vi "VCL_2_DSC_BATCH.vi"(8 "error in (no error)":errorcluster, 11 "path to logfile or directory":path) -> (0 "error out":errorcluster)   [LabVIEW 2016, in "VCL_2_DSC.lvclass"]
uses:
  VCL_2_DSC.lvclass
  typedefs/write-enum.ctl
  <vilib>/addons/WireFlow/_WF_ProgressBar.llb/ProgressBar_WireFlow.lvclass
panel:
  in  "Enum":T1
  in  "Process":bool
  in  "STOP":bool
  out "standard output":string
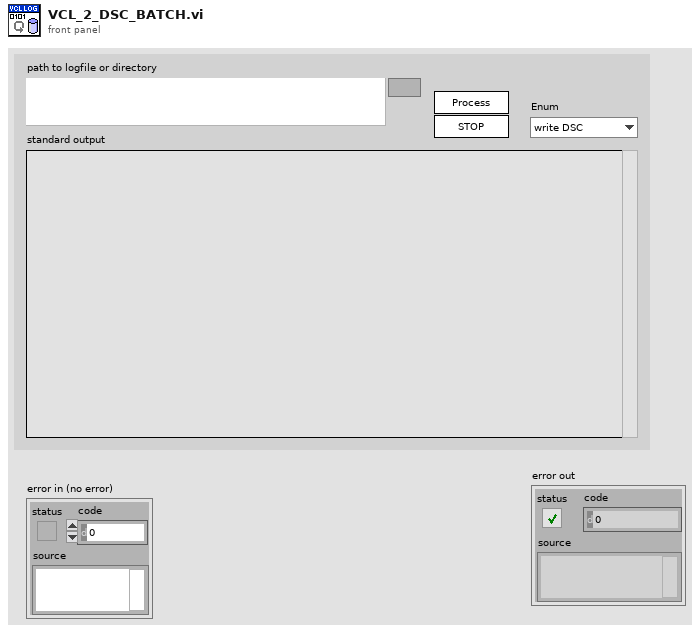
[diagram p1: front panel]
types:
  T1 = typedef "VCL_2_DSC.lvclass/write-enum.ctl" = enum16{"write DSC", "write TDMS", "no write"}
  T2 = enum32{"invalid app kind", "Development System", "Run Time System", "Student Edition", "Embedded LabVIEW", "Evaluation", "Custom"}
  T3 = enum32{"Invalid", "Standard", "Closed", "Hidden", "Minimized", "Maximized"}
  T4 = cluster{"Core":cluster{"Current VI Reference":refnum<vi>, "Close Panel on Exit?":bool}, "vcl paths":path[], "txt paths":path[], "WF-ProgressBar":refnum<class "ProgressBar_WireFlow.lvclass">}
  T5 = cluster{"Current VI Reference":refnum<vi>, "Close Panel on Exit?":bool}
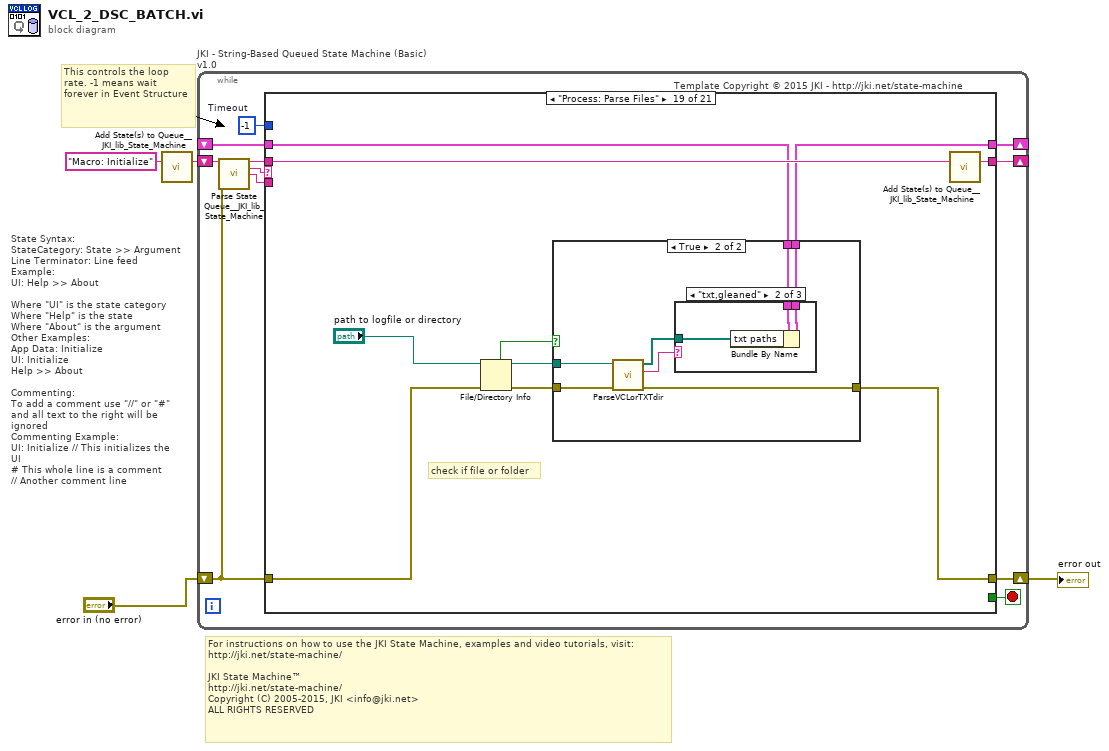
[diagram p0: block diagram]
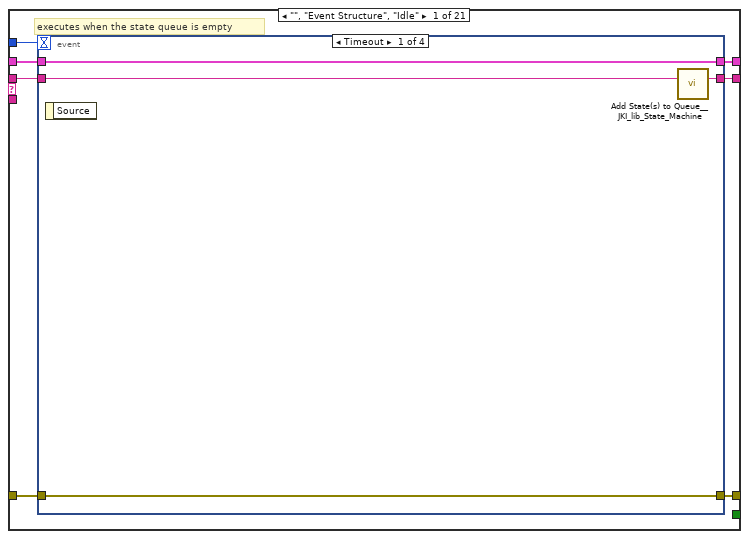
[diagram p2: hidden frame]
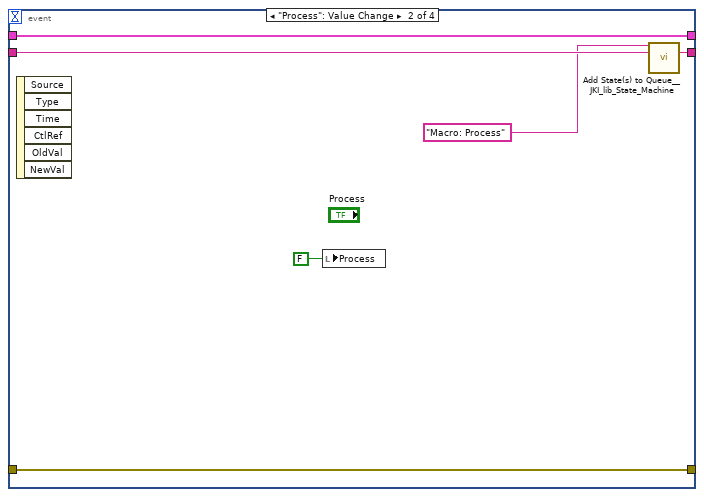
[diagram p3: hidden frame]
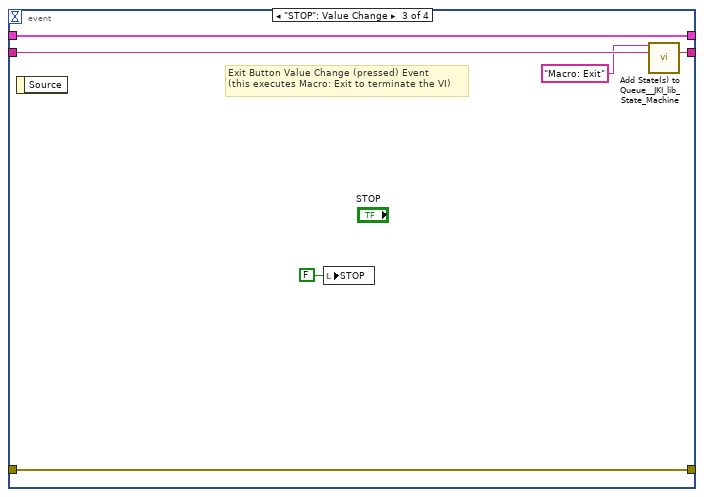
[diagram p4: hidden frame]
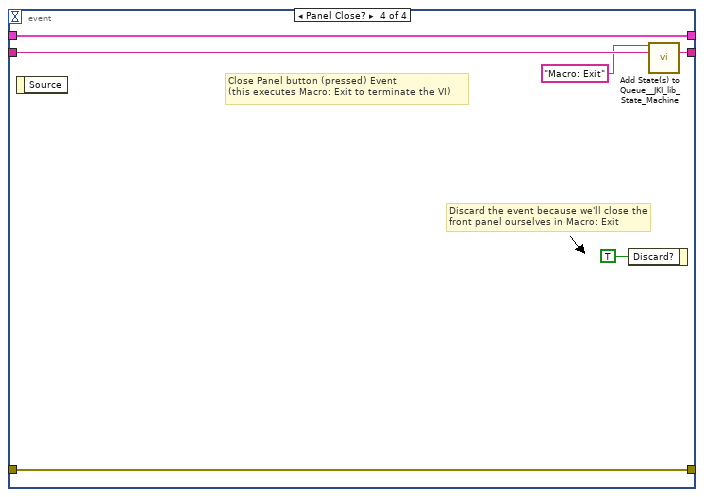
[diagram p5: hidden frame]
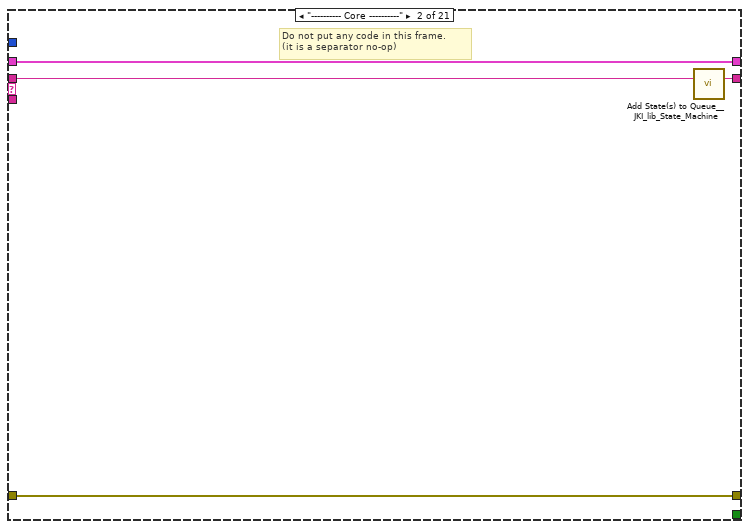
[diagram p6: hidden frame]
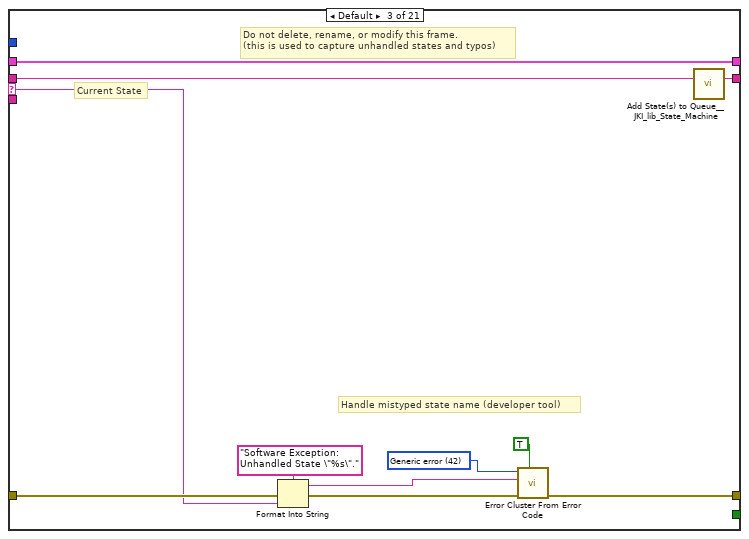
[diagram p7: hidden frame]
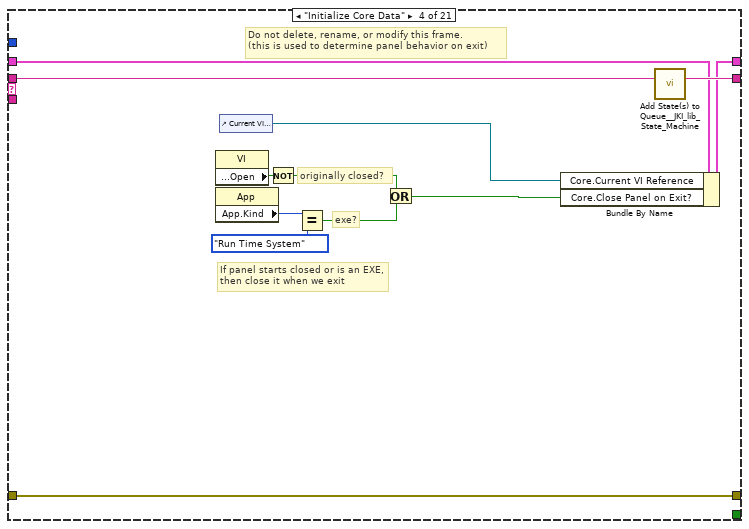
[diagram p8: hidden frame]
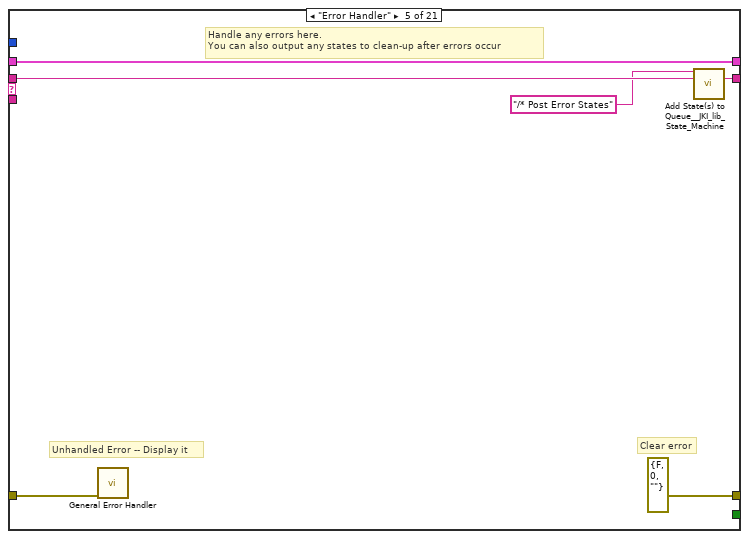
[diagram p9: hidden frame]
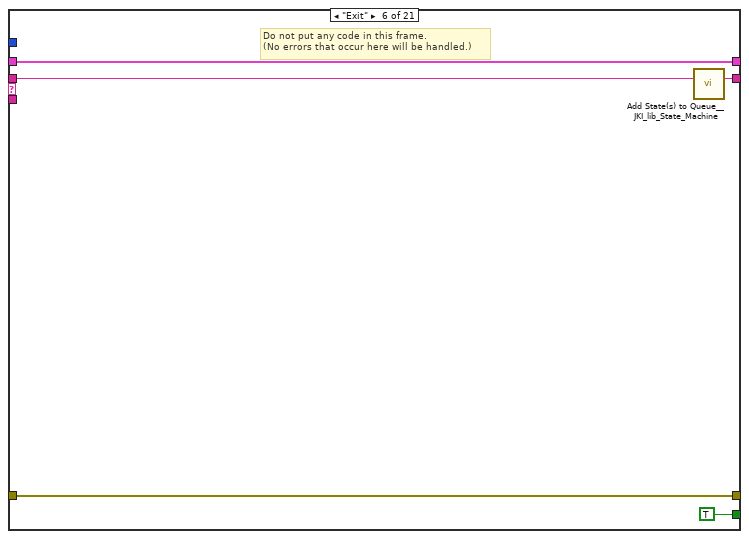
[diagram p10: hidden frame]
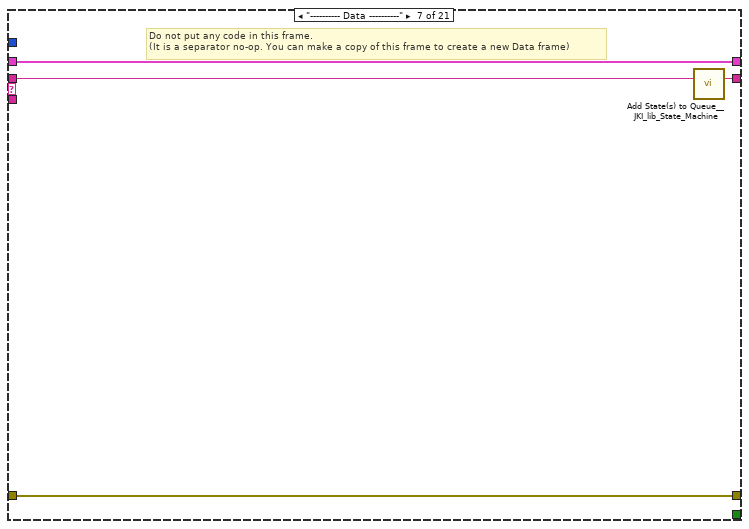
[diagram p11: hidden frame]
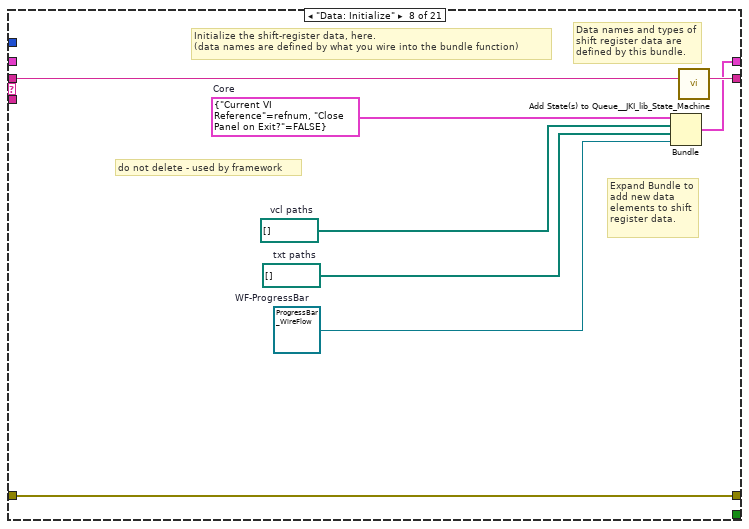
[diagram p12: hidden frame]
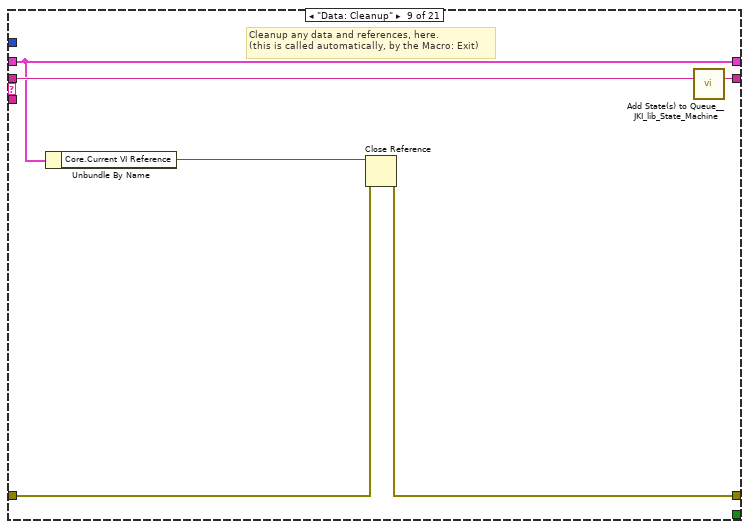
[diagram p13: hidden frame]
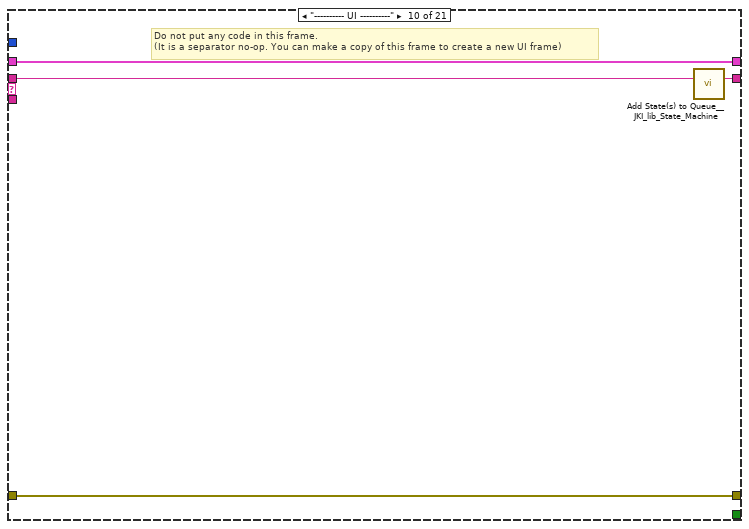
[diagram p14: hidden frame]
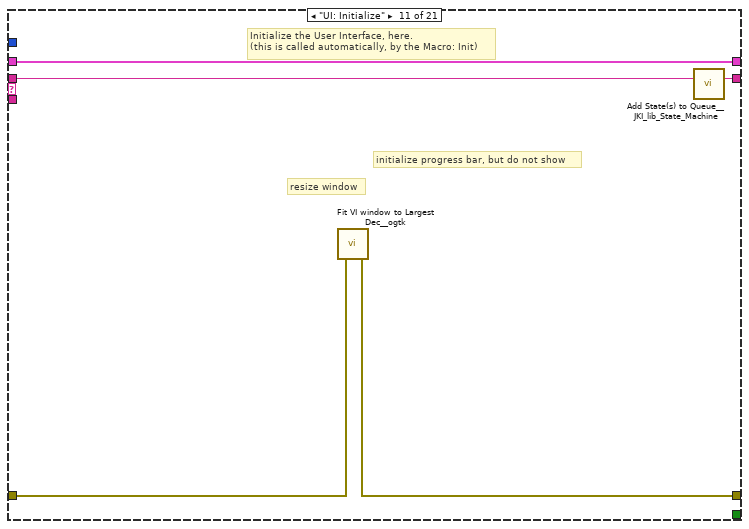
[diagram p15: hidden frame]
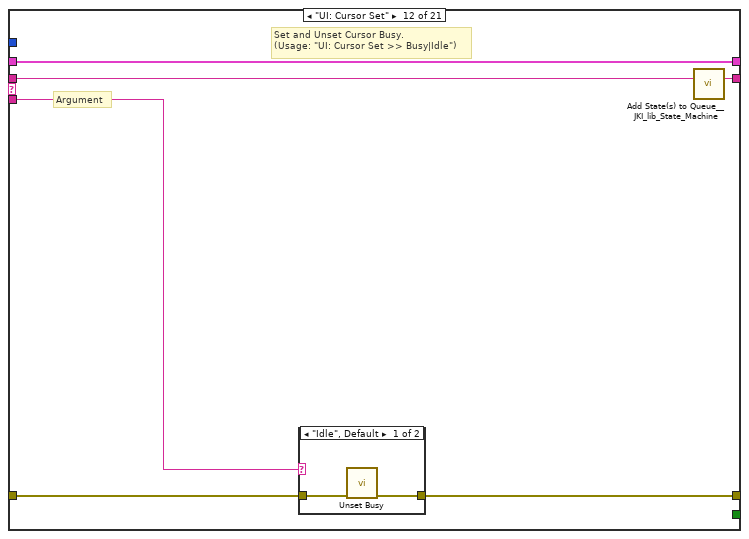
[diagram p16: hidden frame]
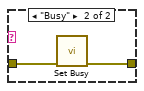
[diagram p17: hidden frame]
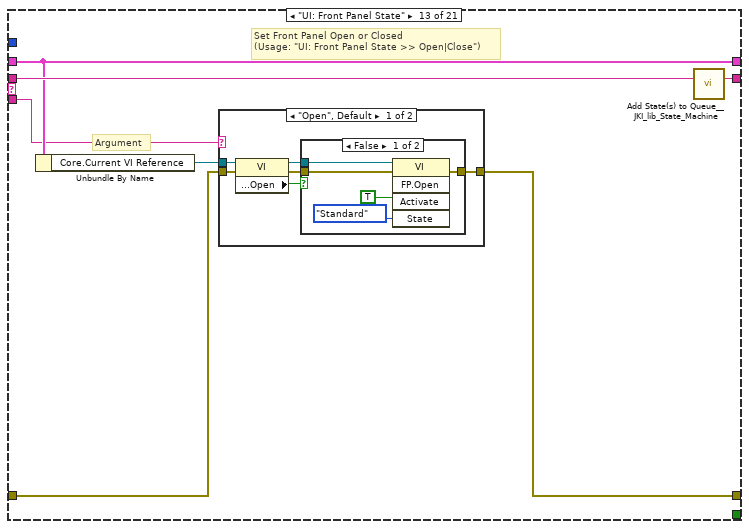
[diagram p18: hidden frame]
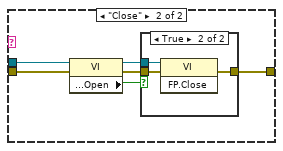
[diagram p20: hidden frame]
diagram:
  # "For instructions on how to use the JKI State Machine, examples and video tutorials, visit:\nhttp://jki.net/state-machine/\n\nJKI State Machine™\nhttp://jki.net/state-machine/\nCopyright (C) 2005-2015, JKI <info@jki.net>\nALL RIGHTS RESERVED"
  # "State Syntax:\nStateCategory: State >> Argument\nLine Terminator: Line feed\nExample:\nUI: Help >> About\n\nWhere \"UI\" is the state category\nWhere \"Help\" is the state\nWhere \"About\" is the argument\nOther Examples:\nApp Data: Initialize\nUI: Initialize\nHelp >> About\n\nCommenting:\nTo add a comment use \"//\" or \"#\" and all text to the right will be ignored\nCommenting Example:\nUI: Initialize // This initializes the UI\n# This whole line is a comment\n// Another comment line"
  # "This controls the loop rate. -1 means wait forever in Event Structure"
  n1 = call <vilib>:"Add State(s) to Queue__JKI_lib_State_Machine.vi"("State(s) in (\"\")"="Macro: Initialize") -> ("States Out"=w4:string)  [unwired: 14 in]
  n2 = while "JKI - String-Based Queued State Machine (Basic) v1.0" {
    shift-right: [w8] -> _
    shift-left: _ -> [w7]
    shift-right: [w11] -> w1
    shift-left: "error in (no error)" -> [w5]
    shift-right: [w10] -> _
    shift-left: w4 -> [w12]
    stop <- w9 stop-if-true
    w6 = -1  # Timeout
    # "Template Copyright © 2015 JKI - http://jki.net/state-machine"
    n3 = call <vilib>:"Parse State Queue__JKI_lib_State_Machine.vi"("State Queue"=w12, "Error In (no error)"=w5) -> ("Remaining States"=w14:string, "Current State"=w15:string, "Arguments"=w13:string)  [unwired: 11 in]
    n4 = case shown="\"Process: Parse Files\"" w15 {
      selector: w15 -> [_ _ w49 _ _ _ _ _ _ _ _ _ _ _ _ _ _ _ _ _ _]
      tunnel: w14 -> [w22 w48 w53 w71 w77 w82 w86 w94 w100 w104 w109 w115 w126 w152 w157 w167 w172 w176 w186 w223 w262]
      tunnel: w13 -> [_ _ _ _ _ _ _ _ _ _ _ w110 w120 _ _ _ _ _ _ _ _]
      tunnel: w7 -> [w20 w45 w51 w62 w74 w80 w83 _ w96 w101 w106 w113 w122 w149 w154 w164 w169 w173 w179 w220 w260]
      tunnel: [w19 w46 w55 w68 errorcluster {"status"=FALSE, "code"=0, "source"=""} ("error out") w79 w84 w91 w97 w102 w105 w111 w123 w150 w155 w165 w170 w174 w180 w217 w257] -> w11
      tunnel: w5 -> [w18 w46 w54 w68 w73 w79 w84 w91 w95 w102 w107 w112 w124 w150 w155 w165 w170 w174 w181 w219 w258]
      tunnel: [w21 w47 w52 w70 w76 w81 w85 w93 w99 w103 w108 w114 w125 w151 w156 w166 w171 w175 w185 w222 w261] -> w10
      tunnel: [_ _ _ _ _ TRUE _ _ _ _ _ _ _ _ _ _ _ _ _ _ _] -> w9
      tunnel: [w17 w45 w51 w69 w74 w80 w83 w92 w96 w101 w106 w113 w122 w149 w154 w164 w169 w173 w178 w221 w259] -> w8
      tunnel: w6 -> [w16 _ _ _ _ _ _ _ _ _ _ _ _ _ _ _ _ _ _ _ _]
      frame "", "Event Structure", "Idle" {
        # "executes when the state queue is empty"
        n5 = event shown="[0] Timeout" {
          selector: _ -> [_ _ _ _]
          dyn-events: _ -> [_ _ _ _]
          timeout: w16 -> [_ _ _ _]
          tunnel: w22 -> [w26 w32 w38 w44]
          tunnel: [w25 w31 w37 w43] -> w21
          tunnel: w20 -> [w23 w29 w35 w41]
          tunnel: [w24 w30 w36 w42] -> w19
          tunnel: w18 -> [w24 w30 w36 w42]
          tunnel: [w23 w29 w35 w41] -> w17
          event Timeout {
            n6 = event-data() -> ()  [unwired: 1 in, 1 out]
            n7 = call <vilib>:"Add State(s) to Queue__JKI_lib_State_Machine.vi"("State(s) in (\"\")"=w26) -> ("States Out"=w25:string)  [unwired: 14 in]
          }
          event "Process": Value Change {
            n8 = event-data() -> ()  [unwired: 1 in, 6 out]
            n9 = local write "Process"(FALSE ("Process")) -> ()
            n10 = call <vilib>:"Add State(s) to Queue__JKI_lib_State_Machine.vi"("State(s) in Front (\"\")"="Macro: Process" ("State(s) in Front (\"\")"), "State(s) in (\"\")"=w32) -> ("States Out"=w31:string)  [unwired: 13 in]
          }
          event "STOP": Value Change {
            # "Exit Button Value Change (pressed) Event\n(this executes Macro: Exit to terminate the VI)"
            n11 = event-data() -> ()  [unwired: 1 in, 1 out]
            n12 = local write "STOP"(FALSE ("STOP")) -> ()
            n13 = call <vilib>:"Add State(s) to Queue__JKI_lib_State_Machine.vi"("State(s) in Front (\"\")"="Macro: Exit", "State(s) in (\"\")"=w38) -> ("States Out"=w37:string)  [unwired: 13 in]
          }
          event Panel Close? {
            # "Discard the event because we'll close the front panel ourselves in Macro: Exit"
            # "Close Panel button (pressed) Event\n(this executes Macro: Exit to terminate the VI)"
            n14 = event-data() -> ()  [unwired: 1 in, 1 out]
            n15 = event-data("Discard?"=TRUE) -> ()  [unwired: 1 in, 1 out]
            n16 = call <vilib>:"Add State(s) to Queue__JKI_lib_State_Machine.vi"("State(s) in Front (\"\")"="Macro: Exit", "State(s) in (\"\")"=w44) -> ("States Out"=w43:string)  [unwired: 13 in]
          }
        }
      }
      frame "---------- Core ----------" {
        # "Do not put any code in this frame.\n(it is a separator no-op)"
        n17 = call <vilib>:"Add State(s) to Queue__JKI_lib_State_Machine.vi"("State(s) in (\"\")"=w48) -> ("States Out"=w47:string)  [unwired: 14 in]
      }
      frame Default {
        w58 = 42 items=["No error", "Argument error", "Memory is full", "Out of zone", "End of file", "File already open", "Generic file I/O error", "File not found", "File permission error", "Disk is full", "Duplicate path", "Too many files open", "System feature not enabled", "Resource file not found", "Cannot add resource", "Resource not found", "Image not found", "Image memory error", "Pen does not exist", "Config type invalid", "Config token not found", "Config parse error", "Config memory error", "Bad external code format", "Bad external code offset", "External code not present", "Null window", "Destroy window error", "Null menu", "Print aborted", "Bad print record", "Print driver error", "Windows error during printing", "Memory error during printing", "Print dialog error", "Generic print error", "Invalid device refnum", "Device not found", "Device parameter error", "Device unit error", "Cannot open device", "Device call aborted", "Generic error", "Cancelled by user", "Object ID too low", "Object ID too high", "Object not in heap", "Unknown heap", "Unknown object (invalid DefProc)", "Unknown object (DefProc not in table)", "Message out of range", "Invalid (null) method", "Unknown message", "Manager call not supported", "Bad address", "Network operation in progress", "Network operation timed out", "Connection is busy", "Network attribute not supported", "Network error", "Address in use", "System out of memory", "Connection aborted", "Connection refused", "Not connected", "Already connected", "Connection closed", "Initialization error (interapplication manager)", "Bad occurrence", "Wait on unbound occurrence handler", "Occurrence queue overflow", "Datalog type conflict", "Unused", "Unrecognized type (interapplication manager)", "Memory corrupt", "Failed to make temporary DLL", "Old CIN version", "Drag socket not found", "Failed to load drop-object", "Failed to register OLE object", "Failed to release OLE object", "Format specifier type mismatch", "Unknown format specifier", "Too few format specifiers", "Too many format specifiers", "Scan failed", "Newer CIN version", "Error converting to variant", "Runtime menu error", "Password tampered", "Variant attribute not found", "Incompatible variant data type", "Event data is not available", "Event Store is not present", "Occurrence is not found", "Event Queue is not created", "Event info is not available", "Refnum passed is NULL", "Error retrieving Class GUID", "Error retrieving CoClass GUID", "Error retrieving TypeLib GUID.", "Bad built application magic bytes.", "Specific driver is different from the specific driver associated with the Logical Name.", "There is no session opened to the class driver.", "Max Error", "MAX - Error with config objects", "MAX - Error loading configuration", "MAX - Group not supported"]
        # "Current State"
        # "Do not delete, rename, or modify this frame.\n(this is used to capture unhandled states and typos)"
        # "Handle mistyped state name (developer tool)"
        n18 = Format Into String(format string="Software Exception: Unhandled State \"%s\"." ("message"), error in=w54, w49) -> (resulting string=w57:string, error out=w56:errorcluster)  [unwired: 1 in]
        n19 = call <vilib>:"Error Cluster From Error Code.vi"("show call chain? (False)"=TRUE, "error in (no error)"=w56, "error message (\"\")"=w57, "error code (0)"=w58) -> ("error out"=w55:errorcluster)  [unwired: 5 in]
        n20 = call <vilib>:"Add State(s) to Queue__JKI_lib_State_Machine.vi"("State(s) in (\"\")"=w53) -> ("States Out"=w52:string)  [unwired: 14 in]
      }
      frame "Initialize Core Data" {
        # "Do not delete, rename, or modify this frame.\n(this is used to determine panel behavior on exit)"
        # "originally closed?"
        # "exe?"
        # "If panel starts closed or is an EXE, then close it when we exit"
        n21 = property class="VI"() -> ("Front Panel.Open"=w67:bool)  [unwired: 2 in, 2 out]
        n22 = property class="App"() -> ("App.Kind"=w66:T2)  [unwired: 2 in, 2 out]
        n23 = control-ref of="Current VI Reference"() -> (w60:refnum<vi>)
        n24 = Not(x=w67) -> (.not. x?=w64:bool)
        n25 = Equal?(x=w66, y=T2."Run Time System" ("Application:Kind")) -> (x = y?=w63:bool)
        n26 = Or(x=w64, y=w63) -> (x .or. y?=w61:bool)
        n27 = Bundle By Name(cluster=w62, "Core.Current VI Reference"=w60, "Core.Close Panel on Exit?"=w61) -> (w69:T4)
        n28 = call <vilib>:"Add State(s) to Queue__JKI_lib_State_Machine.vi"("State(s) in (\"\")"=w71) -> ("States Out"=w70:string)  [unwired: 14 in]
      }
      frame "Error Handler" {
        # "Unhandled Error -- Display it"
        # "Handle any errors here.\nYou can also output any states to clean-up after errors occur"
        # "Clear error"
        n29 = call <vilib>:"General Error Handler.vi"("error in (no error)"=w73) -> ()  [unwired: 10 in, 5 out]
        n30 = call <vilib>:"Add State(s) to Queue__JKI_lib_State_Machine.vi"("State(s) in Front (\"\")"="/* Post Error States", "State(s) in (\"\")"=w77) -> ("States Out"=w76:string)  [unwired: 13 in]
      }
      frame "Exit" {
        # "Do not put any code in this frame.\n(No errors that occur here will be handled.)"
        n31 = call <vilib>:"Add State(s) to Queue__JKI_lib_State_Machine.vi"("State(s) in (\"\")"=w82) -> ("States Out"=w81:string)  [unwired: 14 in]
      }
      frame "---------- Data ----------" {
        # "Do not put any code in this frame.\n(It is a separator no-op. You can make a copy of this frame to create a new Data frame)"
        n32 = call <vilib>:"Add State(s) to Queue__JKI_lib_State_Machine.vi"("State(s) in (\"\")"=w86) -> ("States Out"=w85:string)  [unwired: 14 in]
      }
      frame "Data: Initialize" {
        w87 = path[] []  # txt paths
        w88 = path[] []  # vcl paths
        w89 = refnum<class "ProgressBar_WireFlow.lvclass"> refnum  # WF-ProgressBar
        w90 = T5 {"Current VI Reference"=refnum, "Close Panel on Exit?"=FALSE}  # Core
        # "do not delete - used by framework"
        # "Expand Bundle to add new data elements to shift register data."
        # "Data names and types of shift register data are defined by this bundle."
        # "Initialize the shift-register data, here.\n(data names are defined by what you wire into the bundle function)"
        n33 = Bundle("Core"=w90, "vcl paths"=w88, "txt paths"=w87, "WF-ProgressBar"=w89) -> (w92:T4)  [unwired: 1 in]
        n34 = call <vilib>:"Add State(s) to Queue__JKI_lib_State_Machine.vi"("State(s) in (\"\")"=w94) -> ("States Out"=w93:string)  [unwired: 14 in]
      }
      frame "Data: Cleanup" {
        # "Cleanup any data and references, here.\n(this is called automatically, by the Macro: Exit)"
        n35 = Unbundle By Name(w96) -> ("Core.Current VI Reference"=w98:refnum<vi>)
        n36 = Close Reference(reference=w98, error in (no error)=w95) -> (error out=w97:errorcluster)
        n37 = call <vilib>:"Add State(s) to Queue__JKI_lib_State_Machine.vi"("State(s) in (\"\")"=w100) -> ("States Out"=w99:string)  [unwired: 14 in]
      }
      frame "---------- UI ----------" {
        # "Do not put any code in this frame.\n(It is a separator no-op. You can make a copy of this frame to create a new UI frame)"
        n38 = call <vilib>:"Add State(s) to Queue__JKI_lib_State_Machine.vi"("State(s) in (\"\")"=w104) -> ("States Out"=w103:string)  [unwired: 14 in]
      }
      frame "UI: Initialize" {
        # "initialize progress bar, but do not show"
        # "resize window"
        # "Initialize the User Interface, here.\n(this is called automatically, by the Macro: Init)"
        n39 = call <userlib>:"Fit VI window to Largest Dec__ogtk.vi"("error in (no error)"=w107) -> ("error out"=w105:errorcluster)  [unwired: 5 in, 1 out]
        n40 = call <vilib>:"Add State(s) to Queue__JKI_lib_State_Machine.vi"("State(s) in (\"\")"=w109) -> ("States Out"=w108:string)  [unwired: 14 in]
      }
      frame "UI: Cursor Set" {
        # "Argument"
        # "Set and Unset Cursor Busy.\n(Usage: \"UI: Cursor Set >> Busy|Idle\")"
        n41 = case shown="\"Idle\", Default" w110 {
          tunnel: w112 -> [w117 w119]
          tunnel: [w116 w118] -> w111
          frame "Idle", Default {
            n42 = call <vilib>:"Unset Busy.vi"("error in (no error)"=w117) -> ("error out"=w116:errorcluster)  [unwired: 10 in]
          }
          frame "Busy" {
            n43 = call <vilib>:"Set Busy.vi"("error in (no error)"=w119) -> ("error out"=w118:errorcluster)  [unwired: 9 in, 1 out]
          }
        }
        n44 = call <vilib>:"Add State(s) to Queue__JKI_lib_State_Machine.vi"("State(s) in (\"\")"=w115) -> ("States Out"=w114:string)  [unwired: 14 in]
      }
      frame "UI: Front Panel State" {
        # "Argument"
        # "Set Front Panel Open or Closed\n(Usage: \"UI: Front Panel State >> Open|Close\")"
        n45 = Unbundle By Name(w122) -> ("Core.Current VI Reference"=w121:refnum<vi>)
        n46 = case shown="\"Open\", Default" w120 {
          tunnel: w124 -> [w130 w143]
          tunnel: [w132 w144] -> w123
          tunnel: w121 -> [w131 w141]
          frame "Open", Default {
            n47 = property class="VI"(reference=w131, error in=w130) -> (reference out=w128:refnum<vi>, error out=w129:errorcluster, "Front Panel.Open"=w127:bool)
            n48 = case shown="False" w127 {
              tunnel: [w135 w138] -> w132
              tunnel: w129 -> [w134 w138]
              tunnel: w128 -> [w133 _]
              frame False {
                n49 = invoke class="VI" method="FP.Open"(reference=w133, error in=w134, "Activate"=TRUE, "State"=T3."Standard") -> (error out=w135:errorcluster)  [unwired: 1 in, 4 out]
              }
              frame True {
              }
            }
          }
          frame "Close" {
            n50 = property class="VI"(reference=w141, error in=w143) -> (reference out=w140:refnum<vi>, error out=w142:errorcluster, "Front Panel.Open"=w139:bool)
            n51 = case shown="True" w139 {
              tunnel: [w145 w148] -> w144
              tunnel: w142 -> [w145 w147]
              tunnel: w140 -> [_ w146]
              frame False {
              }
              frame True {
                n52 = invoke class="VI" method="FP.Close"(reference=w146, error in=w147) -> (error out=w148:errorcluster)  [unwired: 1 in, 2 out]
              }
            }
          }
        }
        n53 = call <vilib>:"Add State(s) to Queue__JKI_lib_State_Machine.vi"("State(s) in (\"\")"=w126) -> ("States Out"=w125:string)  [unwired: 14 in]
      }
      frame "---------- Macro ----------" {
        # "Do not put any code in this frame.\n(It is a separator no-op. You can make a copy of this frame to create a new Macro frame)"
        n54 = call <vilib>:"Add State(s) to Queue__JKI_lib_State_Machine.vi"("State(s) in (\"\")"=w152) -> ("States Out"=w151:string)  [unwired: 14 in]
      }
      frame "Macro: Initialize" {
        w153 = "Data: Initialize\nInitialize Core Data\nUI: Initialize\nUI: Front Panel State >> Open"  # Data: Initialize Initialize Core Data UI: Initialize UI: Front Panel State >> Open
        # "Initialization Macro\n(This is called once, when the VI starts)"
        n55 = call <vilib>:"Add State(s) to Queue__JKI_lib_State_Machine.vi"("State(s) in Front (\"\")"=w153, "State(s) in (\"\")"=w157) -> ("States Out"=w156:string)  [unwired: 13 in]
      }
      frame "Macro: Exit" {
        # "Exit Macro\n(This is called once, when the VI exits)"
        n56 = Unbundle By Name(w164) -> ("Core.Close Panel on Exit?"=w163:bool)
        n57 = Select(t="UI: Front Panel State >> Close", s=w163, f="") -> (s? t:f=w160:string)
        n58 = call <vilib>:"Add State(s) to Queue__JKI_lib_State_Machine.vi"("State(s) in (\"\")"=w160, "State(s) at Back (\"\")"="Data: Cleanup\nExit") -> ("States Out"=w158:string)  [unwired: 13 in]
        n59 = call <vilib>:"Add State(s) to Queue__JKI_lib_State_Machine.vi"("State(s) in Front (\"\")"=w158, "State(s) in (\"\")"=w167) -> ("States Out"=w166:string)  [unwired: 13 in]
      }
      frame "Macro: Process" {
        # "Do not put any code in this frame.\n(It is a separator no-op. You can make a copy of this frame to create a new Macro frame)"
        n60 = call <vilib>:"Add State(s) to Queue__JKI_lib_State_Machine.vi"("State(s) in Front (\"\")"="Process: Parse Files\nProcess: Process VCL\nProcess: Write DSC", "State(s) in (\"\")"=w172) -> ("States Out"=w171:string)  [unwired: 13 in]
      }
      frame "---------- Process ----------" {
        # "Template Separator\n(You can make a copy of, or modify, this frame)"
        n61 = call <vilib>:"Add State(s) to Queue__JKI_lib_State_Machine.vi"("State(s) in (\"\")"=w176) -> ("States Out"=w175:string)  [unwired: 14 in]
      }
      frame "Process: Parse Files" {
        # "check if file or folder"
        n62 = File/Directory Info(path="path to logfile or directory", error in=w181) -> (path out=w184:path, directory=w183:bool, error out=w182:errorcluster)  [unwired: 4 out]
        n63 = case shown="True" w183 {
          tunnel: [w192 w206] -> w180
          tunnel: w182 -> [w193 w207]
          tunnel: w184 -> [w194 w208]
          tunnel: w179 -> [w189 w205]
          tunnel: [w188 w204] -> w178
          frame False {
            n64 = call <vilib>:"Get File Extension.vi"("error in (no error)"=w193, "file"=w194) -> ("error out"=w192:errorcluster, "lowercase file extension"=w187:string, "dup file"=w191:path)  [unwired: 5 in, 2 out]
            n65 = Build Array(w191) -> (w190:path[])
            n66 = case shown="\"vcl\"" w187 {
              tunnel: w190 -> [w197 w200 _]
              tunnel: w189 -> [w196 w199 w201]
              tunnel: [w195 w198 w201] -> w188
              frame "vcl" {
                n67 = Bundle By Name(cluster=w196, "vcl paths"=w197) -> (w195:T4)
              }
              frame "txt,gleaned" {
                n68 = Bundle By Name(cluster=w199, "txt paths"=w200) -> (w198:T4)
              }
              frame Default {
              }
            }
          }
          frame True {
            n69 = call "ParseVCLorTXTdir.vi"("error in (no error)"=w207, "path in"=w208) -> ("error out"=w206:errorcluster, "type"=w202:string, "appended path"=w203:path[])  [unwired: 7 in]
            n70 = case shown="\"txt,gleaned\"" w202 {
              tunnel: w203 -> [w211 w214 _]
              tunnel: w205 -> [w210 w213 w215]
              tunnel: [w209 w212 w215] -> w204
              frame "vcl" {
                n71 = Bundle By Name(cluster=w210, "vcl paths"=w211) -> (w209:T4)
              }
              frame "txt,gleaned" {
                n72 = Bundle By Name(cluster=w213, "txt paths"=w214) -> (w212:T4)
              }
              frame Default {
              }
            }
          }
        }
        n73 = call <vilib>:"Add State(s) to Queue__JKI_lib_State_Machine.vi"("State(s) in (\"\")"=w186) -> ("States Out"=w185:string)  [unwired: 14 in]
      }
      frame "Process: Process VCL" {
        n74 = Unbundle By Name(w220) -> ("vcl paths"=w218:path[])
        n75 = Empty Array?(array=w218) -> (empty?=w216:bool)
        n76 = case shown="False" w216 {
          tunnel: [w236 w253] -> w221
          tunnel: w220 -> [w235 w253]
          tunnel: [w231 w254] -> w217
          tunnel: w219 -> [w226 w254]
          tunnel: w218 -> [w225 _]
          frame False {
            # "converts each *.vcl into *.txt in same directory"
            n77 = Array Size(array=w225) -> (size(s)=w224:i32)
            n78 = call <vilib>:"PB_Init.vi"("error in (no error)"=w226) -> ("error out"=w228:errorcluster, "WF-ProgressBar out"=w227:refnum<class "ProgressBar_WireFlow.lvclass">)  [unwired: 9 in]
            n79 = call-dynamic "SetRangeMinMax.vi"("error in (no error)"=w228, "Max (1)"=w224, "WF-ProgressBar in"=w227) -> ("error out"=w233:errorcluster, "WF-ProgressBar out"=w232:refnum<class "ProgressBar_WireFlow.lvclass">)  [unwired: 7 in]
            n80 = for {
              tunnel: w233 -> [w246]
              tunnel: w225 -> [w252] mode=indexing
              tunnel: w232 -> [w243]
              tunnel: [w250] -> w230
              tunnel: [w249] -> w237 mode=indexing
              tunnel: [w248] -> w229
              tunnel: w224 -> [w239]
              i -> [w247]
              stop <- w244 stop-if-true
              n81 = Increment(x=w247) -> (x+1=w240:i32)
              n82 = Format Into String(format string="converting *.vcl file %1$d of %2$d" ("Message"), error in=w246, w240, w239) -> (resulting string=w242:string, error out=w241:errorcluster)  [unwired: 1 in]
              n83 = call-dynamic "SetProgressMessage.vi"("error in (no error)"=w241, "Progress value (NaN no update)"=w240, "Message"=w242, "WF-ProgressBar in"=w243) -> ("error out"=w251:errorcluster, "WF-ProgressBar out"=w250:refnum<class "ProgressBar_WireFlow.lvclass">)  [unwired: 5 in, 1 out]
              n84 = call "VCL_2_TSV.vi"("error in (no error)"=w251, "Path to VCL file"=w252) -> ("error out"=w248:errorcluster, "standard output"=→"standard output":string, "path to txt file"=w249:path)  [unwired: 7 in]
              n85 = local read "STOP"() -> (w244:bool)
            }
            n86 = call-dynamic "PB_Clear.vi"("error in (no error)"=w229, "WF-ProgressBar in"=w230) -> ("error out"=w231:errorcluster)  [unwired: 8 in, 1 out]
            n87 = Bundle By Name(cluster=w235, "vcl paths"=path[] [], "txt paths"=w237) -> (w236:T4)
          }
          frame True {
          }
        }
        n88 = call <vilib>:"Add State(s) to Queue__JKI_lib_State_Machine.vi"("State(s) in (\"\")"=w223) -> ("States Out"=w222:string)  [unwired: 14 in]
      }
      frame "Process: Write DSC" {
        n89 = Unbundle By Name(w260) -> ("txt paths"=w256:path[])
        n90 = Empty Array?(array=w256) -> (empty?=w255:bool)
        n91 = case shown="False" w255 {
          tunnel: w260 -> [w275 w291]
          tunnel: [w274 w291] -> w259
          tunnel: w258 -> [w267 w290]
          tunnel: [w265 w290] -> w257
          tunnel: w256 -> [w263 _]
          frame False {
            # "converts each *.vcl into *.txt in same directory"
            n92 = Array Size(array=w263) -> (size(s)=w264:i32)
            n93 = call <vilib>:"PB_Init.vi"("error in (no error)"=w267) -> ("error out"=w268:errorcluster, "WF-ProgressBar out"=w266:refnum<class "ProgressBar_WireFlow.lvclass">)  [unwired: 9 in]
            n94 = call-dynamic "SetRangeMinMax.vi"("error in (no error)"=w268, "Max (1)"=w264, "WF-ProgressBar in"=w266) -> ("error out"=w271:errorcluster, "WF-ProgressBar out"=w272:refnum<class "ProgressBar_WireFlow.lvclass">)  [unwired: 7 in]
            n95 = for {
              N -> [w277]
              tunnel: w271 -> [w288]
              tunnel: w263 -> [w285] mode=indexing
              tunnel: w272 -> [w283]
              tunnel: [w289] -> w269
              tunnel: [w287] -> w270
              i -> [w280]
              stop <- w284 stop-if-true
              n96 = Increment(x=w280) -> (x+1=w278:i32)
              n97 = Format Into String(format string="writing to DSC file %1$d of %2$d" ("Message"), error in=w288, w278, w277) -> (resulting string=w282:string, error out=w281:errorcluster)  [unwired: 1 in]
              n98 = local read "STOP"() -> (w284:bool)
              n99 = call-dynamic "SetProgressMessage.vi"("error in (no error)"=w281, "Progress value (NaN no update)"=w278, "Message"=w282, "WF-ProgressBar in"=w283) -> ("error out"=w286:errorcluster, "WF-ProgressBar out"=w289:refnum<class "ProgressBar_WireFlow.lvclass">)  [unwired: 5 in, 1 out]
              n100 = call "TSV_2_DSC.vi"("error in (no error)"=w286, "Enum"="Enum", "path to txt file"=w285) -> ("error out"=w287:errorcluster)  [unwired: 8 in]
            }
            n101 = call-dynamic "PB_Clear.vi"("error in (no error)"=w270, "WF-ProgressBar in"=w269) -> ("error out"=w265:errorcluster)  [unwired: 8 in, 1 out]
            n102 = Bundle By Name(cluster=w275, "txt paths"=path[] []) -> (w274:T4)
          }
          frame True {
          }
        }
        n103 = call <vilib>:"Add State(s) to Queue__JKI_lib_State_Machine.vi"("State(s) in (\"\")"=w262) -> ("States Out"=w261:string)  [unwired: 14 in]
      }
    }
  }
  "error out" <- w1
